vi "MH_DatatoRecMH150T2.vi"(10 "channel":u32, 11 "Time":u32) -> (3 "rawbits":u32)   [LabVIEW 2019]
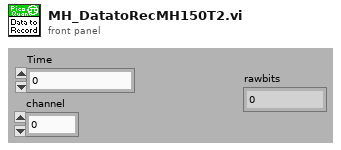
[diagram p1: front panel]
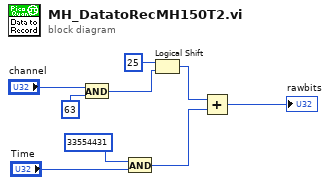
[diagram p0: block diagram]
diagram:
  n1 = And(x="channel", y=u32 63 ("x")) -> (x .and. y?=w5:u32)
  n2 = And(x=u32 33554431, y="Time") -> (x .and. y?=w1:u32)
  n3 = Logical Shift(y=i16 25, x=w5) -> (x << y=w3:u32)
  n4 = Add(x=w3, y=w1) -> (x+y=→"rawbits":u32)
